vi "Read Attributes.vi"(11 "B_msg Msg":refnum<class "B_msg Msg.lvclass">) -> (2 "Payload":cluster{"Status":string})   [LabVIEW 2025, in "B_Actor.lvlib" / "B_msg Msg.lvclass"]
uses:
  B_msg Msg.lvclass
  B_msg Msg.lvclass/B_msg Msg.ctl
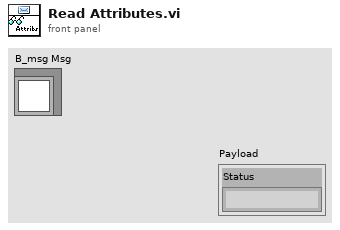
[diagram p1: front panel]
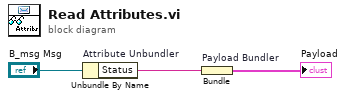
[diagram p0: block diagram]
diagram:
  n1 = Unbundle By Name "Attribute Unbundler"("B_msg Msg") -> ("Status"=w1:string)
  n2 = Bundle "Payload Bundler"("Status"=w1) -> (→"Payload":cluster{"Status":string})  [unwired: 1 in]
